vi "testujPunkty.vi"(9 "Punkty":i32[][](array[numeric]), 10 "Minimalna odległość":dbl=0.7 format="%#_13g", 11 "Promień [m]":dbl=1.0 format="%#_13g") -> (3 "Odleglosci":T1[][](array[typedef]) {"Odległość [m]" format="%#.2g"})   [LabVIEW 2014]
uses:
  testujPunktyVIs/Odleglosc.ctl
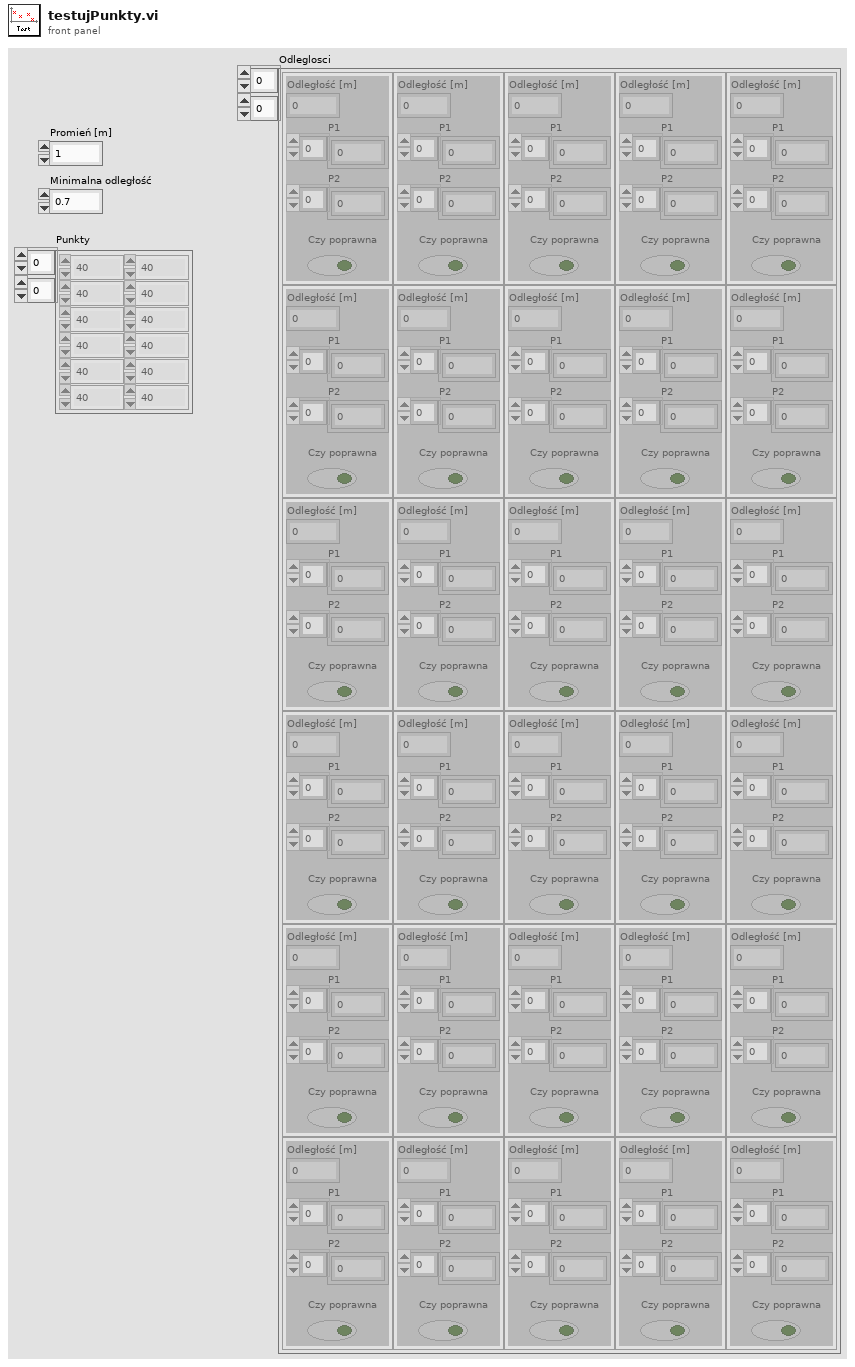
[diagram p1: front panel]
types:
  T1 = typedef "Odleglosc.ctl" = cluster{"Odległość [m]":dbl, "P1":i32[], "P2":i32[], "Czy poprawna":bool}
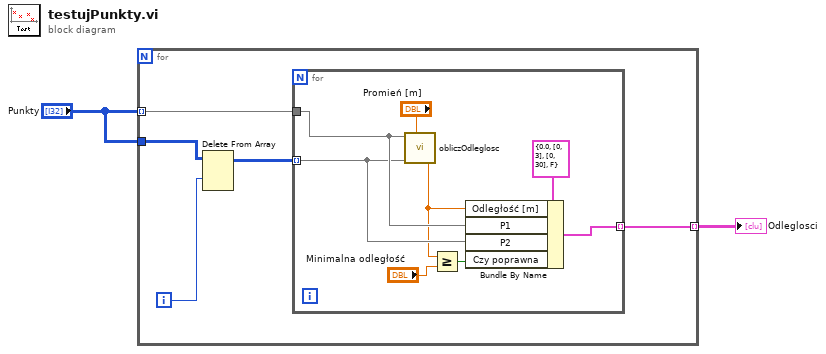
[diagram p0: block diagram]
diagram:
  n1 = for {
    tunnel: "Punkty" -> [w4] mode=indexing
    tunnel: "Punkty" -> [w7]
    tunnel: [w3] -> w1 mode=indexing
    i -> [w6]
    n2 = Delete From Array(array=w7, index (row)=w6) -> (array with subset deleted=w5:i32[][])  [unwired: 2 in, 1 out]
    n3 = for {
      tunnel: w5 -> [w12] mode=indexing
      tunnel: w4 -> [w13]
      tunnel: [w11] -> w3 mode=indexing
      n4 = call "obliczOdleglosc.vi"("Promień [m]"="Promień [m]", "P2"=w12, "P1"=w13) -> ("Odległość [m]"=w9:dbl)  [unwired: 8 in]
      n5 = Greater Or Equal?(x=w9, y="Minimalna odległość") -> (x >= y?=w10:bool)
      n6 = Bundle By Name(cluster=T1 {"Odległość [m]"=0.0, "P1"=[0, 3], "P2"=[0, 30], "Czy poprawna"=FALSE}, "Odległość [m]"=w9, "P1"=w13, "P2"=w12, "Czy poprawna"=w10) -> (w11:T1)
    }
  }
  "Odleglosci" <- w1
